vi "Obtain.vi"(8 "error in (no error)":errorcluster, 9 "create if not found? (T)":bool=TRUE, 10 "Name (\"\")":string, 11 "Notifier in":refnum<class "Notifier.lvclass">) -> (0 "error out":errorcluster, 1 "created new?":bool, 3 "Notifier out":refnum<class "Notifier.lvclass">)   [LabVIEW 2020, in "Data.lvlib" / "Notifier.lvclass"]
doc: "Obtain a Data notifier for the Notifier class."
uses:
  Notifier.lvclass
  Data.lvclass
  Notifier.lvclass/Notifier.ctl
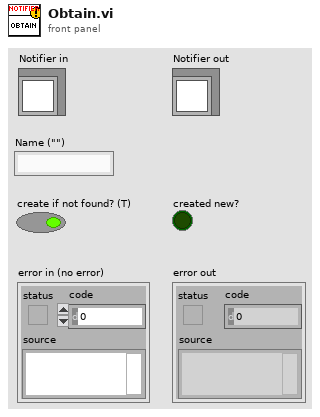
[diagram p1: front panel]
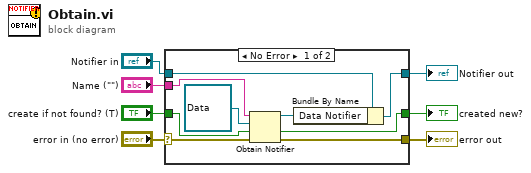
[diagram p0: block diagram]
diagram:
  n1 = case shown="No Error" "error in (no error)" {
    selector: "error in (no error)" -> [w12 w18]
    tunnel: [w11 w18] -> w6
    tunnel: [w14 w17] -> w4
    tunnel: "Notifier in" -> [w16 w17]
    tunnel: "Name (\"\")" -> [w10 _]
    tunnel: "create if not found? (T)" -> [w9 _]
    tunnel: [w8 _] -> w1
    frame No Error {
      n2 = Obtain Notifier(name (unnamed)=w10, notification data type=refnum<class "Data.lvclass"> refnum ("Data.lvlib:Data.lvclass"), create if not found? (T)=w9, error in (no error)=w12) -> (notifier out=w13:refnum<notifier>, created new?=w8:bool, error out=w11:errorcluster)
      n3 = Bundle By Name(cluster=w16, "Data Notifier"=w13) -> (w14:refnum<class "Notifier.lvclass">)
    }
    frame Error {
    }
  }
  "error out" <- w6
  "Notifier out" <- w4
  "created new?" <- w1
